vi "GUID Lookup.vi"() -> ()   [LabVIEW 2019, in "Ghost Bus Addon Shared.lvlib"]
doc: "Use this Global VI to access the GUIDs assigned to the page resources of the Custom Device."
uses:
  Ghost Bus Addon Shared.lvlib
panel:
  in  "Override Channel Page Name":string="Override"
  in  "Data Channel Page Name":string="Data"
  in  "Override Frames Page Name":string="Override Frames"
  in  "Override Frames GUID":string="6DBD21E7-9AC1-4A33-BA91-2620717C270E"
  in  "On Compile Settings":string="On Compile Settings"
  in  "Override Signal GUID":string="A0DBE684-75DE-40FF-ABFB-257FA9974665"
  in  "Data Signal GUID":string="10435930-D9E5-4765-86ED-FFE3B81430E0"
  in  "Frame.ID":string="XNET.Primary.LoopPriority"
  in  "XNET.Ghost.FDISOMode":string="XNET.Ghost.FDISOMode"
  in  "XNET.Ghost.LoopPriority":string="XNET.Ghost.LoopPriority"
  in  "XNET.Ghost.IOMode":string="XNET.Ghost.IOMode"
  in  "XNET.Ghost.FDRate":string="XNET.Ghost.FDRate"
  in  "XNET.Ghost.Termination":string="XNET.Ghost.Termination"
  in  "XNET.Ghost.Rate":string="XNET.Ghost.Rate"
  in  "XNET.Ghost.Port":string="XNET.Ghost.Port"
  in  "To Primary Bus Page Name":string="To Primary Bus"
  in  "To Ghost Bus Page Name":string="To Ghost Bus"
  in  "Settings Page Name":string="Settings"
  in  "Enable Page Name":string="Enable"
  in  "Enable Channel GUID":string="6B6F940E-5E79-447D-84E5-02DD399E6370"
  in  "Settings GUID":string="9EFE9432-3035-4F22-AD7D-DDC55D3B893F"
  in  "To Primary Bus GUID":string="F56B78C2-8EF9-4685-942E-B770392E4C5B"
  in  "To Ghost Bus GUID":string="7467F215-F187-4AC4-A182-357DF27361BD"
  in  "Override Frame GUID":string="3D195969-2661-40C8-A580-19595CD6B5C5"
  in  "Status Channel GUID":string="1C67F462-1B2F-4305-AD9C-25DD02EFA2E8"
  in  "Status GUID":string="8E6559CC-D8D1-4FEC-967E-A75255AC33F0"
  in  "Status Page Name":string="Status"
  in  "Status.Duration":string="Duration"
  in  "Status.ErrorStatus":string="Error Code"
  in  "Status.Period":string="Period"
  in  "XNET.Primary.FDISOMode":string="XNET.Primary.FDISOMode"
  in  "XNET.Primary.LoopPriority":string="XNET.Primary.LoopPriority"
  in  "XNET.Primary.IOMode":string="XNET.Primary.IOMode"
  in  "XNET.Primary.FDRate":string="XNET.Primary.FDRate"
  in  "XNET.Primary.Termination":string="XNET.Primary.Termination"
  in  "XNET.Primary.Rate":string="XNET.Primary.Rate"
  in  "XNET.Primary.Port":string="XNET.Primary.Port"
  in  "XNET.Cluster":string="XNET.Cluster"
  in  "XNET.Database":string="XNET.Database"
  in  "Help.FileName":string="Ghost Bus Addon.chm"
  out "Error Codes":cluster{"number":i32, "trimmed string":string}[](array[cluster])=[{"number"=0, "trimmed string"="<0> No Error."}, {"number"=-1074384895, "trimmed string"="<-1074384895> An internal error occurred in the NI-XNET driver."}, {"number"=-1074384894, "trimmed string"="<-1074384894> Board self test failed(code 2)."}, {"number"=-1074384893, "trimmed string"="<-1074384893> Board self test failed(code 3)."}, {"number"=-1074384892, "trimmed string"="<-1074384892> Board self test failed(code 4)."}, {"number"=-1074384891, "trimmed string"="<-1074384891> Board self test failed(code 5)."}, {"number"=-1074384890, "trimmed string"="<-1074384890> Board self test failed(code 6)."}, {"number"=-1074384889, "trimmed string"="<-1074384889> Computer went to hibernation mode and the board lost power."}, {"number"=-1074384888, "trimmed string"="<-1074384888> A write queue overflowed."}, {"number"=-1074384887, "trimmed string"="<-1074384887> The board's firmware did not answer a command."}, {"number"=-1074384886, "trimmed string"="<-1074384886> The operation timed out."}, {"number"=-1074384885, "trimmed string"="<-1074384885> A read queue overflowed."}, {"number"=-1074384884, "trimmed string"="<-1074384884> The Read buffer is too small to hold a single frame."}, {"number"=-1074384883, "trimmed string"="<-1074384883> You tried to open the same frame twice."}, {"number"=-1074384882, "trimmed string"="<-1074384882> You tried to open the same stream object twice."}, {"number"=-1074384881, "trimmed string"="<-1074384881> Self test is not possible since the board is in use by an application."}, {"number"=-1074384880, "trimmed string"="<-1074384880> Allocation of memory failed."}, {"number"=-1074384879, "trimmed string"="<-1074384879> The maximum number of sessions was exceeded."}, {"number"=-1074384878, "trimmed string"="<-1074384878> The maximum number of sessions has been exceeded."}, {"number"=-1074384877, "trimmed string"="<-1074384877> The maximum number of devices has been detected."}, {"number"=-1074384876, "trimmed string"="<-1074384876> A driver support file is missing."}, {"number"=-1074384875, "trimmed string"="<-1074384875> This indicates that a NULL pointer or an empty string was passed to a function."}, {"number"=-1074384874, "trimmed string"="<-1074384874> The maximum number of schedules has been detected."}, {"number"=-1074384873, "trimmed string"="<-1074384873> Board self test failed (code 17)."}, {"number"=-1074384872, "trimmed string"="<-1074384872> You cannot start an NI-XNET application while a self test is in progress."}, {"number"=-1074384864, "trimmed string"="<-1074384864> An invalid reference has been passed to a NI-XNET session function."}, {"number"=-1074384863, "trimmed string"="<-1074384863> An invalid reference has been passed to a NI-XNET system function."}, {"number"=-1074384862, "trimmed string"="<-1074384862> A device reference was expected for a NI-XNET session function."}, {"number"=-1074384861, "trimmed string"="<-1074384861> An interface reference was expected for a NI-XNET session function."}, {"number"=-1074384860, "trimmed string"="<-1074384860> You have configured a property that conflicts with the current mode of the session."}, {"number"=-1074384859, "trimmed string"="<-1074384859> The XNET Create Timing Source VI is supported only on LabVIEW Real-Time targets currently running the Phar Lap ETS Real-Time Operating System."}, {"number"=-1074384858, "trimmed string"="<-1074384858> You tried to create more than one LabVIEW timing source for a single interface."}, {"number"=-1074384857, "trimmed string"="<-1074384857> You invoked two or more VIs simultaneously for the same session, and those VIs do not support overlap."}, {"number"=-1074384856, "trimmed string"="<-1074384856> You are trying to start an interface that is missing bus power for the transceiver."}, {"number"=-1074384855, "trimmed string"="<-1074384855> The connection with a CompactDAQ chassis was lost, and the host software and modules are out of sync."}, {"number"=-1074384783, "trimmed string"="<-1074384783> The transceiver value set is invalid (for this port, e.g., LS on a HS port) or you are trying to perform an operation that requires a different transceiver (e.g., trying to change the state of a disconnected transceiver)."}, {"number"=-1074384782, "trimmed string"="<-1074384782> The baud rate value set is invalid."}, {"number"=-1074384781, "trimmed string"="<-1074384781> No baud rate value has been set."}, {"number"=-1074384780, "trimmed string"="<-1074384780> The bit timing values set are invalid."}, {"number"=-1074384779, "trimmed string"="<-1074384779> The baud rate set does not match the transceiver's allowed range."}, {"number"=-1074384778, "trimmed string"="<-1074384778> The configured terminal is not known for this interface."}, {"number"=-1074384777, "trimmed string"="<-1074384777> The configured terminal is inappropriate for the hardware."}, {"number"=-1074384776, "trimmed string"="<-1074384776> The source that you connected to the Master Timebase destination is missing."}, {"number"=-1074384775, "trimmed string"="<-1074384775> The source that you connected to the Master Timebase destination is not generating an appropriate signal."}, {"number"=-1074384774, "trimmed string"="<-1074384774> You are trying to disconnect a synchronization terminal that is not currently connected."}, {"number"=-1074384773, "trimmed string"="<-1074384773> You are trying to connect a synchronization terminal that is already in use."}, {"number"=-1074384772, "trimmed string"="<-1074384772> You are trying to connect an XNET terminal as a source terminal,  but the desired XNET terminal is not valid as a source terminal."}, {"number"=-1074384771, "trimmed string"="<-1074384771> You are trying to connect an XNET terminal as a destination terminal, but the desired XNET terminal is not valid as a destination terminal."}, {"number"=-1074384770, "trimmed string"="<-1074384770> You are trying to connect two XNET terminals that are incompatible."}, {"number"=-1074384769, "trimmed string"="<-1074384769> The source that you connected to the Master Timebase destination has disappeared."}, {"number"=-1074384768, "trimmed string"="<-1074384768> You called Read (State : FlexRay : Cycle Macrotick), and the FlexRay Macrotick is not connected as the master timebase of the interface."}, {"number"=-1074384767, "trimmed string"="<-1074384767> The database specified could not be opened."}, {"number"=-1074384766, "trimmed string"="<-1074384766> The cluster was not found in the database."}, {"number"=-1074384765, "trimmed string"="<-1074384765> The frame was not found in the database."}, {"number"=-1074384764, "trimmed string"="<-1074384764> The signal was not found in the database."}, {"number"=-1074384763, "trimmed string"="<-1074384763> A necessary property for a cluster was not found in the database."}, {"number"=-1074384762, "trimmed string"="<-1074384762> A necessary property for a frame was not found in the database."}, {"number"=-1074384761, "trimmed string"="<-1074384761> A necessary property for a signal was not found in the database."}, {"number"=-1074384760, "trimmed string"="<-1074384760> Multiple clusters have been specified in one session, either directly (Stream I/O), or through the signals or frames specified."}, {"number"=-1074384759, "trimmed string"="<-1074384759> You specified a database of ':subordinate:' for a session mode other than mode of Frame Input Stream."}, {"number"=-1074384758, "trimmed string"="<-1074384758> The interface name given does not specify a valid and existing interface."}, {"number"=-1074384757, "trimmed string"="<-1074384757> The operation is invalid for this interface (e.g., you tried to open a set of FlexRay frames on a CAN interface, or tried to request a CAN property from a FlexRay interface)."}, {"number"=-1074384756, "trimmed string"="<-1074384756> You tried to set the AutoStart property to FALSE for an Input session."}, {"number"=-1074384755, "trimmed string"="<-1074384755> The property ID you specified is not valid (or not valid for the current session mode or form factor)."}, {"number"=-1074384754, "trimmed string"="<-1074384754> The contents of the property is bigger than the size specified."}, {"number"=-1074384753, "trimmed string"="<-1074384753> The function you called is not defined for the session mode (e.g., you called a frame I/O function on a signal I/O session)."}, {"number"=-1074384752, "trimmed string"="<-1074384752> The data that you passed to XNET Write or XNET Read is too small to hold all the data specified for the session."}, {"number"=-1074384751, "trimmed string"="<-1074384751> For Signal Output sessions, the multiplexer signals used in the session must be specified explicitly in the signal list."}, {"number"=-1074384750, "trimmed string"="<-1074384750> You used an XNET Session IO name, and that session was not found in your LabVIEW project."}, {"number"=-1074384749, "trimmed string"="<-1074384749> You used the same XNET session name in multiple top-level VIs, which is not supported."}, {"number"=-1074384748, "trimmed string"="<-1074384748> To execute this function properly, the session's list must contain only one frame."}, {"number"=-1074384747, "trimmed string"="<-1074384747> You used the same alias for different database files which is not allowed."}, {"number"=-1074384746, "trimmed string"="<-1074384746> You try to deploy a database file while another deployment is in progress."}, {"number"=-1074384745, "trimmed string"="<-1074384745> A signal or frame session has been opened, but it does not contain signals or frames."}, {"number"=-1074384744, "trimmed string"="<-1074384744> The session mode selected is not supported by the protocol of the specified interface."}, {"number"=-1074384743, "trimmed string"="<-1074384743> A session was created by references, but no database references have been specified."}, {"number"=-1074384742, "trimmed string"="<-1074384742> The interface has already been opened with different cluster settings than the ones specified for this session."}, {"number"=-1074384741, "trimmed string"="<-1074384741> The cycle repetition of a frame in the database for the FlexRay protocol is invalid."}, {"number"=-1074384740, "trimmed string"="<-1074384740> You called XNET Clear for the session, then tried to perform another operation."}, {"number"=-1074384739, "trimmed string"="<-1074384739> You called Create Session VI with a list of items that does not match the mode."}, {"number"=-1074384738, "trimmed string"="<-1074384738> You tried to create a new session while the interface is already running."}, {"number"=-1074384737, "trimmed string"="<-1074384737> You wrote a frame whose payload length is larger than the maximum payload allowed by the database (e.g., wrote 10 bytes for CAN frame, max 8 bytes)."}, {"number"=-1074384736, "trimmed string"="<-1074384736> You called a Read function with a nonzero timeout, and you used a negative numberToRead."}, {"number"=-1074384735, "trimmed string"="<-1074384735> Timestamps are not (yet) supported for Write Signal XY."}, {"number"=-1074384734, "trimmed string"="<-1074384734> The condition parameter passed to Wait is not known."}, {"number"=-1074384733, "trimmed string"="<-1074384733> You attempted an I/O operation, but the session is not yet started (and the AutoStart property is set to FALSE)."}, {"number"=-1074384732, "trimmed string"="<-1074384732> The maximum number of Wait operations has been exceeded."}, {"number"=-1074384731, "trimmed string"="<-1074384731> You used an invalid name for an XNET Device."}, {"number"=-1074384730, "trimmed string"="<-1074384730> A terminal name passed to ConnectTerminals or DisconnectTerminals is unknown."}, {"number"=-1074384729, "trimmed string"="<-1074384729> You tried to blink the port LEDs but these are currently busy."}, {"number"=-1074384728, "trimmed string"="<-1074384728> You tried to set a FlexRay keyslot ID that is not listed as valid in the database."}, {"number"=-1074384727, "trimmed string"="<-1074384727> You tried to set a queue size that is bigger than the maximum allowed."}, {"number"=-1074384726, "trimmed string"="<-1074384726> You wrote a frame whose payload length is different than the payload length configured by the database."}, {"number"=-1074384725, "trimmed string"="<-1074384725> The index to indicate an session list element is too large."}, {"number"=-1074384724, "trimmed string"="<-1074384724> You have tried to create a session that is invalid for the mode of the driver/firmware."}, {"number"=-1074384723, "trimmed string"="<-1074384723> The trigger signal for a frame is allowed only in Single Point Signal sessions (Input or Output)."}, {"number"=-1074384722, "trimmed string"="<-1074384722> To execute this function properly, the session's list must contain only one cluster."}, {"number"=-1074384721, "trimmed string"="<-1074384721> You attempted to convert a CAN or LIN frame with a payload length greater than 8."}, {"number"=-1074384720, "trimmed string"="<-1074384720> Allocation of memory failed for the data returned from LabVIEW XNET Read."}, {"number"=-1074384719, "trimmed string"="<-1074384719> Allocation of memory failed in the firmware."}, {"number"=-1074384718, "trimmed string"="<-1074384718> The NI-XNET driver no longer can communicate with the device."}, {"number"=-1074384717, "trimmed string"="<-1074384717> A LIN schedule has an invalid priority."}, {"number"=-1074384716, "trimmed string"="<-1074384716> (Dis)ConnectTerminals is not allowed for XNET C Series modules."}, {"number"=-1074384715, "trimmed string"="<-1074384715> You requested a time (like Start or Communication Time) before the event has happened."}, {"number"=-1074384714, "trimmed string"="<-1074384714> An internal input queue overflowed."}, {"number"=-1074384713, "trimmed string"="<-1074384713> A bad firmware image file can not be loaded to the hardware."}, {"number"=-1074384712, "trimmed string"="<-1074384712> The encoding of embedded network data (CAN, FlexRay, LIN, etc.) within the TDMS file is invalid."}, {"number"=-1074384711, "trimmed string"="<-1074384711> The NI-XNET hardware no longer can communicate with the transceiver cable."}, {"number"=-1074384710, "trimmed string"="<-1074384710> The NI-XNET driver timed out when performing low-level communication with the device."}, {"number"=-1074384709, "trimmed string"="<-1074384709> A transfer to the C Series module was aborted."}, {"number"=-1074384708, "trimmed string"="<-1074384708> An invalid value has been specified for the CAN FD ISO Mode."}, {"number"=-1074384704, "trimmed string"="<-1074384704> A property value was out of range or incorrect."}, {"number"=-1074384703, "trimmed string"="<-1074384703> Integration of the interface into the FlexRay cluster failed, so communication did not start for the interface."}, {"number"=-1074384688, "trimmed string"="<-1074384688> The PDU was not found in the database."}, {"number"=-1074384687, "trimmed string"="<-1074384687> A necessary property for a PDU was not found in the database."}, {"number"=-1074384686, "trimmed string"="<-1074384686> You tried to open the same PDU twice."}, {"number"=-1074384685, "trimmed string"="<-1074384685> You can access this database object only by PDU, not by frame."}, {"number"=-1074384640, "trimmed string"="<-1074384640> Remote communication with the LabVIEW RT target failed."}, {"number"=-1074384639, "trimmed string"="<-1074384639> File transfer communication with the LabVIEW Real-Time (RT) target failed."}, {"number"=-1074384638, "trimmed string"="<-1074384638> File transfer to the LabVIEW Real-Time (RT) target failed, because the required files could not be accessed."}, {"number"=-1074384637, "trimmed string"="<-1074384637> The database file you want to use is already assigned to another alias."}, {"number"=-1074384636, "trimmed string"="<-1074384636> An internal file used by NI-XNET could not be accessed."}, {"number"=-1074384635, "trimmed string"="<-1074384635> The file cannot be deployed because another file deployment is already active."}, {"number"=-1074384617, "trimmed string"="<-1074384617> The nixnet.dll or one of its components could not be loaded."}, {"number"=-1074384610, "trimmed string"="<-1074384610> You attempted to perform an action on a session or interface that is started, and the action that requires the session/interface to be stopped."}, {"number"=-1074384609, "trimmed string"="<-1074384609> You have passed a default payload to the firmware where the number of bytes in the payload is larger than the number of bytes that this frame can transmit."}, {"number"=-1074384605, "trimmed string"="<-1074384605> You attempted to set a CAN arbitration ID with an invalid value."}, {"number"=-1074384604, "trimmed string"="<-1074384604> You attempted to set a LIN ID with an invalid value."}, {"number"=-1074384592, "trimmed string"="<-1074384592> Too many open files."}, {"number"=-1074384591, "trimmed string"="<-1074384591> Bad reference has been passed to a database function, e.g., a session reference, or frame reference to retrieve properties from a signal."}, {"number"=-1074384590, "trimmed string"="<-1074384590> Creating a database file failed."}, {"number"=-1074384589, "trimmed string"="<-1074384589> A cluster with the same name already exists in the database."}, {"number"=-1074384588, "trimmed string"="<-1074384588> A frame with the same name already exists in the cluster."}, {"number"=-1074384587, "trimmed string"="<-1074384587> A signal with the same name already exists in the frame."}, {"number"=-1074384586, "trimmed string"="<-1074384586> An ECU with the same name already exists in the cluster."}, {"number"=-1074384585, "trimmed string"="<-1074384585> A subframe with the same name already exists in the frame."}, {"number"=-1074384584, "trimmed string"="<-1074384584> The operation is improper for the protocol in use, e.g., you cannot assign FlexRay channels to a CAN frame."}, {"number"=-1074384583, "trimmed string"="<-1074384583> Wrong parent relationship for a child that you are creating with XNET Database Create."}, {"number"=-1074384581, "trimmed string"="<-1074384581> The retrieved required property is not defined on the specified object."}, {"number"=-1074384580, "trimmed string"="<-1074384580> The feature is not supported under LabVIEW RT, e.g.Save Database"}, {"number"=-1074384579, "trimmed string"="<-1074384579> The object name contains unsupported characters."}, {"number"=-1074384578, "trimmed string"="<-1074384578> Unsupported database format."}, {"number"=-1074384577, "trimmed string"="<-1074384577> Database object not found (e.g., an object with given name does not exist)."}, {"number"=-1074384576, "trimmed string"="<-1074384576> Database cache file cannot be removed or replaced on the disc (e.g., file is write-protected)."}, {"number"=-1074384575, "trimmed string"="<-1074384575> You are trying to write a read-only property, e.g., the mux value on a signal is a read only property (can be changed on the subframe)."}, {"number"=-1074384574, "trimmed string"="<-1074384574> You are trying to change a signal to be a mux signal, but a mux is already defined in this frame"}, {"number"=-1074384572, "trimmed string"="<-1074384572> You are trying to define FlexRay in-cycle-repetition slots before defining the first slot."}, {"number"=-1074384571, "trimmed string"="<-1074384571> You are trying to define FlexRay in-cycle-repetition channels before defining the first channels."}, {"number"=-1074384570, "trimmed string"="<-1074384570> You must define the protocol before setting this property (e.g., the frame ID has a different meaning in a CAN or FlexRay cluster)."}, {"number"=-1074384569, "trimmed string"="<-1074384569> The database information on the real-time system has been created with an older NI-XNET version."}, {"number"=-1074384568, "trimmed string"="<-1074384568> Frame ConfigStatus: A signal within the frame exceeds the frame boundaries (Payload Length)."}, {"number"=-1074384567, "trimmed string"="<-1074384567> Frame ConfigStatus: A signal within the frame overlaps another signal."}, {"number"=-1074384566, "trimmed string"="<-1074384566> Frame ConfigStatus: A integer signal within the frame is defined with more than 52 bits."}, {"number"=-1074384565, "trimmed string"="<-1074384565> Frame ConfigStatus: Frame is defined with an invalid payload size."}, {"number"=-1074384564, "trimmed string"="<-1074384564> You are trying to add transmitted FlexRay frames to an ECU, with at least two of them having Startup or Sync property on."}, {"number"=-1074384563, "trimmed string"="<-1074384563> You are trying to add TX/RX frames to an ECU which are defined in a different cluster than the ECU."}, {"number"=-1074384562, "trimmed string"="<-1074384562> Database name parameter is incorrect."}, {"number"=-1074384561, "trimmed string"="<-1074384561> Database object is locked because it is used in a session."}, {"number"=-1074384560, "trimmed string"="<-1074384560> Alias name passed to a function is not defined."}, {"number"=-1074384559, "trimmed string"="<-1074384559> Database file cannot be saved because frames are assigned to FlexRay channels not defined in the cluster."}, {"number"=-1074384558, "trimmed string"="<-1074384558> Frame ConfigStatus: This FlexRay frame transmitted in a dynamic segment uses both channels A and B."}, {"number"=-1074384557, "trimmed string"="<-1074384557> Database is locked because it is being modified by an another instance of the same application."}, {"number"=-1074384556, "trimmed string"="<-1074384556> A frame name is ambiguous (e.g., a frame with the same name exists in another cluster)."}, {"number"=-1074384555, "trimmed string"="<-1074384555> A signal name is ambiguous (e.g., a signal with the same name exists in another frame)."}, {"number"=-1074384554, "trimmed string"="<-1074384554> An ECU name is ambiguous (e.g., an ECU with the same name exists in another cluster)."}, {"number"=-1074384553, "trimmed string"="<-1074384553> A subframe name is ambiguous (e.g., a subframe with the same name exists in another cluster)."}, {"number"=-1074384552, "trimmed string"="<-1074384552> A LIN schedule name is ambiguous (e.g., a schedule with the same name exists in another cluster)."}, {"number"=-1074384551, "trimmed string"="<-1074384551> A LIN schedule with the same name already exists in the database."}, {"number"=-1074384550, "trimmed string"="<-1074384550> Multiplexers (mode-dependent signals) are not supported when the given protocol is used."}, {"number"=-1074384549, "trimmed string"="<-1074384549> Saving a FIBEX file containing a LIN cluster is not supported in this NI-XNET version."}, {"number"=-1074384548, "trimmed string"="<-1074384548> This property requires an ECU configured as LIN master to be present in this cluster."}, {"number"=-1074384547, "trimmed string"="<-1074384547> You have tried to create a session using a frame that is incompatible with the selected session type."}, {"number"=-1074384546, "trimmed string"="<-1074384546> You cannot mix open of NI-XNET database objects as both manual and automatic."}, {"number"=-1074384545, "trimmed string"="<-1074384545> Due to problems in LabVIEW versions 8.5 through 8.6.1, automatic open of NI-XNET database objects is not supported."}, {"number"=-1074384544, "trimmed string"="<-1074384544> You called a Write function with the number of array elements (frames or signals) different than the number of elements configured in the session (such as the \"list\" parameter of the Create Session function)."}, {"number"=-1074384543, "trimmed string"="<-1074384543> You used XNET session from multiple LabVIEW projects (or multiple executables), which NI-XNET does not support."}, {"number"=-1074384542, "trimmed string"="<-1074384542> When an XNET session is used at runtime, all sessions in the same scope are created on the interface."}, {"number"=-1074384541, "trimmed string"="<-1074384541> You used an empty name for an XNET database object (database, cluster, ECU, frame, or signal)."}, {"number"=-1074384540, "trimmed string"="<-1074384540> You used a name for an XNET database object (such as frame or signal) that did not include a valid cluster selection."}, {"number"=-1074384539, "trimmed string"="<-1074384539> Unsupported database file version."}, {"number"=-1074384538, "trimmed string"="<-1074384538> You used an empty name for the XNET Session."}, {"number"=-1074384537, "trimmed string"="<-1074384537> There is not enough message RAM on the FlexRay hardware to configure the data partition for the object(s)."}, {"number"=-1074384536, "trimmed string"="<-1074384536> The FlexRay keyslot ID has been configured and a startup session has been created."}, {"number"=-1074384535, "trimmed string"="<-1074384535> An unsupported session was created."}, {"number"=-1074384528, "trimmed string"="<-1074384528> An XNET session was created after starting the Interface."}, {"number"=-1074384527, "trimmed string"="<-1074384527> The Single Slot property was enabled on the XNET FlexRay Interface after the interface had started."}, {"number"=-1074384526, "trimmed string"="<-1074384526> The FlexRay macrotick offset specified for XNET Create Timing Source is unsupported."}, {"number"=-1074384525, "trimmed string"="<-1074384525> You used invalid syntax in the name of a database object (signal, frame, or ECU)."}, {"number"=-1074384524, "trimmed string"="<-1074384524> A LIN schedule entry name is ambiguous, e.g., a schedule entry with the same name exists in another schedule."}, {"number"=-1074384523, "trimmed string"="<-1074384523> A LIN schedule entry with the same name already exists in the schedule."}, {"number"=-1074384522, "trimmed string"="<-1074384522> At least one of the frames in the session has an undefined identifier."}, {"number"=-1074384521, "trimmed string"="<-1074384521> At least one of the frames in the session has an undefined payload length."}, {"number"=-1074384520, "trimmed string"="<-1074384520> At least one of the signals in the session has an undefined start bit."}, {"number"=-1074384519, "trimmed string"="<-1074384519> At least one of the signals in the session has an undefined number of bits."}, {"number"=-1074384518, "trimmed string"="<-1074384518> At least one of the signals in the session has an undefined byte order."}, {"number"=-1074384517, "trimmed string"="<-1074384517> At least one of the signals in the session has an undefined data type."}, {"number"=-1074384516, "trimmed string"="<-1074384516> At least one of the subframes in the session has an undefined multiplexer value."}, {"number"=-1074384515, "trimmed string"="<-1074384515> You provided an invalid index to Write (State LIN Schedule Change)."}, {"number"=-1074384514, "trimmed string"="<-1074384514> You provided an invalid name to Write (State LIN Schedule Change)."}, {"number"=-1074384513, "trimmed string"="<-1074384513> You provided an invalid active index for the session property.\nFor LabVIEW, this is the Frame:Active in the session property node.\nFor C/C++, this is the ActiveIndex parameter of nxGetSubProperty/nxSetSubProperty."}, {"number"=-1074384512, "trimmed string"="<-1074384512> You provided an invalid name for Frame:Active of the session property node."}, {"number"=-1074384511, "trimmed string"="<-1074384511> The database you are using requires using PDUs, and the operation is ambiguous with respect to PDUs."}, {"number"=-1074384510, "trimmed string"="<-1074384510> A PDU with the same name already exists in the cluster."}, {"number"=-1074384509, "trimmed string"="<-1074384509> You are trying to assign start bits or update bits to PDUs referenced in a frame, but the number of elements in this array is different than the number of referenced PDUs."}, {"number"=-1074384508, "trimmed string"="<-1074384508> The configuration of this object requires using advanced PDUs, which the given protocol does not support."}, {"number"=-1074384507, "trimmed string"="<-1074384507> The maximum number of PDUs has been exceeded."}, {"number"=-1074384506, "trimmed string"="<-1074384506> This mode value is not currently supported."}, {"number"=-1074384505, "trimmed string"="<-1074384505> The firmware image on your XNET hardware is corrupted."}, {"number"=-1074384504, "trimmed string"="<-1074384504> The firmware version of your XNET hardware is not in sync with your host computer."}, {"number"=-1074384503, "trimmed string"="<-1074384503> The firmware version of your XNET C Series module is not in sync with the NI-XNET software on your remote target."}, {"number"=-1074384502, "trimmed string"="<-1074384502> The terminal you are trying to use is already in use."}, {"number"=-1074384501, "trimmed string"="<-1074384501> You need to install a supported version of NI-DAQmx for your XNET C Series module to work correctly with your Compact DAQ system."}, {"number"=-1074384500, "trimmed string"="<-1074384500> Unable to create the requested route."}, {"number"=-1074384499, "trimmed string"="<-1074384499> You attempted to transmit a go to sleep frame (by setting the LIN Sleep mode to Remote Sleep) on a LIN interface configured as slave."}, {"number"=-1074384498, "trimmed string"="<-1074384498> You attempted to set properties related to Sleep and Wakeup when the FlexRay cluster defined in the Fibex file does not support it."}, {"number"=-1074384497, "trimmed string"="<-1074384497> A LIN diagnostic schedule change requires the diagnostic schedule to be defined in the database."}, {"number"=-1074384494, "trimmed string"="<-1074384494> The data payload written for a diagnostic frame for transmit does not conform to the LIN transport layer specification."}, {"number"=-1074384493, "trimmed string"="<-1074384493> An error occurred within the NI-XNET example code for logfile access (TDMS)."}, {"number"=-1074384384, "trimmed string"="<-1074384384> You attempted to write a LIN schedule and use a stream output replay timing mode concurrently."}, {"number"=-1074384383, "trimmed string"="<-1074384383> You attempted to create a session that is incompatible with the LIN interface personality (master or slave), or set the LIN interface personality to one that is incompatible with a session already created for it."}, {"number"=-1074384382, "trimmed string"="<-1074384382> You attempted to save an LDF or DBC database, but the passed reference is not a database cluster."}, {"number"=-1074384381, "trimmed string"="<-1074384381> You tried to assign the same interface name twice."}, {"number"=-1074384380, "trimmed string"="<-1074384380> Transceiver cable hardware revision is too new."}, {"number"=-1074384379, "trimmed string"="<-1074384379> Transceiver cable image revision is too new."}, {"number"=-1074384378, "trimmed string"="<-1074384378> The property does not apply to this type of hardware."}, {"number"=-1074384377, "trimmed string"="<-1074384377> Exporting cluster into the specified database type failed."}, {"number"=-1074384376, "trimmed string"="<-1074384376> A J1939 input queue overflowed."}, {"number"=-1074384375, "trimmed string"="<-1074384375> You are trying to transmit a non-J1939 frame with more than 8 bytes."}, {"number"=-1074384374, "trimmed string"="<-1074384374> You are trying to transmit a J1939 frame, but no J1939 address is assigned to the session."}, {"number"=-1074384373, "trimmed string"="<-1074384373> The received J1939 TP.CM_CTS message has the wrong total size."}, {"number"=-1074384372, "trimmed string"="<-1074384372> The next packet value of the received J1939 TP.CM_CTS message is larger than the total number of packets."}, {"number"=-1074384371, "trimmed string"="<-1074384371> The received J1939 TP.CM_CTS message has a number of packets of 0, but the next packet number is not 255."}, {"number"=-1074384370, "trimmed string"="<-1074384370> The received J1939 TP.CM_CTS message has a next packet value of 0."}, {"number"=-1074384369, "trimmed string"="<-1074384369> The received J1939 TP.CM_CTS message does not have the same PGN as in the TP.CM_RTS message."}, {"number"=-1074384368, "trimmed string"="<-1074384368> Received unexpected sequence number in the J1939 TP.DT message."}, {"number"=-1074384367, "trimmed string"="<-1074384367> More Packets are requested than allowed in the J1939 TP.CM_CTS message."}, {"number"=-1074384366, "trimmed string"="<-1074384366> J1939 Timeout T1 while waiting for data."}, {"number"=-1074384365, "trimmed string"="<-1074384365> J1939 Timeout T2 while waiting for data."}, {"number"=-1074384364, "trimmed string"="<-1074384364> J1939 Timeout T3 while waiting for TP.CM_CTS or TP.CM_EndOfMsgAck."}, {"number"=-1074384363, "trimmed string"="<-1074384363> J1939 Timeout T4 while waiting for next CTS MSG."}, {"number"=-1074384362, "trimmed string"="<-1074384362> Received wrong DLC in the J1939 TP.CM_RTS message."}, {"number"=-1074384361, "trimmed string"="<-1074384361> Received wrong DLC in the J1939 TP.CM_CTS message."}, {"number"=-1074384360, "trimmed string"="<-1074384360> Received wrong DLC in the J1939 TP.CM_BAM message."}, {"number"=-1074384359, "trimmed string"="<-1074384359> Received wrong DLC in the J1939 TP.DT message."}, {"number"=-1074384358, "trimmed string"="<-1074384358> Received wrong DLC in the J1939 TP.CM_Abort message."}, {"number"=-1074384357, "trimmed string"="<-1074384357> Received wrong DLC in the J1939 TP.CM_EndOfMsgAck message."}, {"number"=-1074384356, "trimmed string"="<-1074384356> Received wrong PGN in the J1939 TP.CM_Abort message."}, {"number"=-1074384355, "trimmed string"="<-1074384355> Internal error occurred for send TP.CM_CTS Hold Message."}, {"number"=-1074384354, "trimmed string"="<-1074384354> Invalid total message size in J1939 TP.CM_RTS message."}, {"number"=-1074384353, "trimmed string"="<-1074384353> Total number of packets in received J1939 TP.CM_RTS message must be greater than 1."}, {"number"=-1074384352, "trimmed string"="<-1074384352> Reserved data bytes in J1939 received message are not BFF63FF."}, {"number"=-1074384351, "trimmed string"="<-1074384351> Not enough system resources for the J1939 Transport Protocol."}, {"number"=-1074384350, "trimmed string"="<-1074384350> Received J1939 TP.CM_Abort message with reason ActiveConnection: Already in one or more connection managed sessions and cannot support another."}, {"number"=-1074384349, "trimmed string"="<-1074384349> Received J1939 TP.CM_Abort message with reason NotEnoughSystemResources: System resources were needed for another task, so this connection managed session was terminated."}, {"number"=-1074384348, "trimmed string"="<-1074384348> Received J1939 TP.CM_Abort message with reason Timeout: A timeout occurred, and this is the connection abort to close the session."}, {"number"=-1074384347, "trimmed string"="<-1074384347> Received J1939 TP.CM_Abort message with reason CtsReceived: CTS messages received when data transfer is in progress."}, {"number"=-1074384346, "trimmed string"="<-1074384346> Received J1939 TP.CM_Abort message with reason MaxRetransmit: Maximum retransmit request limit reached."}, {"number"=-1074384345, "trimmed string"="<-1074384345> Remote communication with the LabVIEW RT target failed because the host and target versions of NI-XNET are different."}, {"number"=-1074384344, "trimmed string"="<-1074384344> The CAN frame I/O mode is higher than the CAN cluster  I/O mode."}, {"number"=-1074384343, "trimmed string"="<-1074384343> The current driver cannot update the firmware on your hardware."}, {"number"=-1074384342, "trimmed string"="<-1074384342> You are trying to use the CAN Transmit I/O Mode (TxIoMode) property in an unsupported interface mode."}, {"number"=-1074384341, "trimmed string"="<-1074384341> You are trying to use the XS Transceiver Cable on unsupported hardware."}, {"number"=-1074384340, "trimmed string"="<-1074384340> You are trying to use a database alias name that contains an invalid character (for example, a comma)."}, {"number"=-1074384339, "trimmed string"="<-1074384339> You are trying to use a database filepath that contains an invalid character (for example, a comma)."}, {"number"=-1074384338, "trimmed string"="<-1074384338> You are trying to use CAN FD with a non-HS/FD port."}, {"number"=-1074384337, "trimmed string"="<-1074384337> An unconditional LIN schedule entry is incorrectly configured."}, {"number"=-1074384336, "trimmed string"="<-1074384336> An event LIN schedule entry has no collision resolving schedule assigned."}, {"number"=-1074384335, "trimmed string"="<-1074384335> You have connected your USB device to a port that supports only Full Speed (USB 1.1)."}, {"number"=-1074384334, "trimmed string"="<-1074384334> You added two or more frames with different payload sizes to the same LIN event-triggered schedule entry."}, {"number"=-1074384333, "trimmed string"="<-1074384333> You added two or more frames with different checksum types to the same event-triggered schedule entry."}, {"number"=-1074384332, "trimmed string"="<-1074384332> The versions of the NI-XNET device driver and Compact RIO driver are incompatible."}, {"number"=-1074384331, "trimmed string"="<-1074384331> The module support for this slot is missing features required for the NI-XNET driver to be able to communicate with the module."}, {"number"=-1074384330, "trimmed string"="<-1074384330> The interface you have attempted to use with NI-XNET Compatibility Library is already in use by NI-XNET."}, {"number"=-1074384329, "trimmed string"="<-1074384329> The interface you have attempted to use with NI-XNET is already in use by NI-XNET Compatibility Library."}, {"number"=-1074384328, "trimmed string"="<-1074384328> Byte array signals are not allowed for this session type or function."}, {"number"=-1074384327, "trimmed string"="<-1074384327> Mixing of byte array signals and numeric signals is not allowed for this session type."}, {"number"=-1074384326, "trimmed string"="<-1074384326> Only one byte array signal is allowed for this session type or function."}, {"number"=-1074384325, "trimmed string"="<-1074384325> The feature you have attempted to use is not supported."}, {"number"=-1074384324, "trimmed string"="<-1074384324> The specified property is write-only and is therefore not readable."}, {"number"=-1074384323, "trimmed string"="<-1074384323> FPGA download is not possible because the board is in use by an application."}, {"number"=-1074384322, "trimmed string"="<-1074384322> The trigger timestamp cannot be read, because the trigger source is not connected."}, {"number"=-1074384321, "trimmed string"="<-1074384321> The trigger timestamp cannot be read, because another operation is reading the timestamp."}, {"number"=-1074384320, "trimmed string"="<-1074384320> The wait did not complete, because it was aborted."}, {"number"=-1074384319, "trimmed string"="<-1074384319> The future time trigger cannot be generated, because the trigger destination is not connected."}, {"number"=-1074384318, "trimmed string"="<-1074384318> The log file could not be created because it already exists."}, {"number"=-1074384317, "trimmed string"="<-1074384317> Could not create or replace the log file."}, {"number"=-1074384316, "trimmed string"="<-1074384316> You cannot read data using XNET Read after a session has been started with logging enabled."}, {"number"=-1074384315, "trimmed string"="<-1074384315> A problem has been detected with the firmware on the device."}, {"number"=-1074384314, "trimmed string"="<-1074384314> A write queue overflowed for a session that has not been started."}, {"number"=-1074384313, "trimmed string"="<-1074384313> The total size of the data to be transmitted is larger than the internal write queue."}, {"number"=-1074384312, "trimmed string"="<-1074384312> The requested number of packets do not fit in the current queue."}, {"number"=-1074384311, "trimmed string"="<-1074384311> You wrote a frame whose payload length is smaller than the minimum payload size allowed."}, {"number"=-1074384310, "trimmed string"="<-1074384310> The XNET endpoint on this port cannot start while the Port Mode is set to Tap."}, {"number"=-1074384309, "trimmed string"="<-1074384309> The future time trigger cannot be generated because a previously scheduled future time trigger is still pending."}, {"number"=-1074384308, "trimmed string"="<-1074384308> The desired time to generate the future time trigger has already elapsed."}, {"number"=-1074384307, "trimmed string"="<-1074384307> The network time cannot be adjusted while this clock is a slave (i.e., not grandmaster)."}, {"number"=-1074384306, "trimmed string"="<-1074384306> Output sessions must be created using an interface's endpoint path."}, {"number"=-1074384305, "trimmed string"="<-1074384305> The time protocol cannot be used while the Port Mode is set to Tap."}, {"number"=-1074384304, "trimmed string"="<-1074384304> You cannot write data while the XNET session is started and the link is down."}, {"number"=-1074384303, "trimmed string"="<-1074384303> Device reset is not possible since the board is in use by an application."}, {"number"=-1074384302, "trimmed string"="<-1074384302> You cannot start an NI-XNET application while a device reset is in progress."}, {"number"=-1074384301, "trimmed string"="<-1074384301> You wrote a frame whose frame type value is not valid."}, {"number"=-1074384300, "trimmed string"="<-1074384300> The data path you have attempted to use is already in use by another session."}, {"number"=-1074384299, "trimmed string"="<-1074384299> The timescale value is invalid."}, {"number"=-1074384298, "trimmed string"="<-1074384298> A hardware error has occurred while reading the Port MAC address."}, {"number"=-1074384297, "trimmed string"="<-1074384297> You cannot write to the Time Sync Protocol property while the Port Mode is set to Tap."}, {"number"=-1074384296, "trimmed string"="<-1074384296> The buffer is not large enough to contain the requested path."}, {"number"=-1074384295, "trimmed string"="<-1074384295> A NULL pointer or an empty string was passed when requesting a path."}, {"number"=1073098816, "trimmed string"="<1073098816> The CAN FD baud rate you supplied exceeds the capabilities the transceiver manufacturer specified."}, {"number"=1073098885, "trimmed string"="<1073098885> There is a warning from importing the database file."}, {"number"=1073098886, "trimmed string"="<1073098886> The database file has been imported, but it was not created by the XNET Editor or using the XNET API."}, {"number"=1073098887, "trimmed string"="<1073098887> The database file was not created by the XNET Editor or using the XNET API."}, {"number"=1073099057, "trimmed string"="<1073099057> Close Database returns a warning instead of an error when an invalid reference is passed to the function."}, {"number"=1073099058, "trimmed string"="<1073099058> You are retrieving signals from a frame that uses advanced PDU configuration."}]
  in  "Custom Device GUID_Disabled":string="FAA7F77A-E3DD-4739-BD52-E4C14A9D9572"
  in  "Custom Device GUID":string="F665F79A-31C5-4337-8154-8A722BDBE03B"
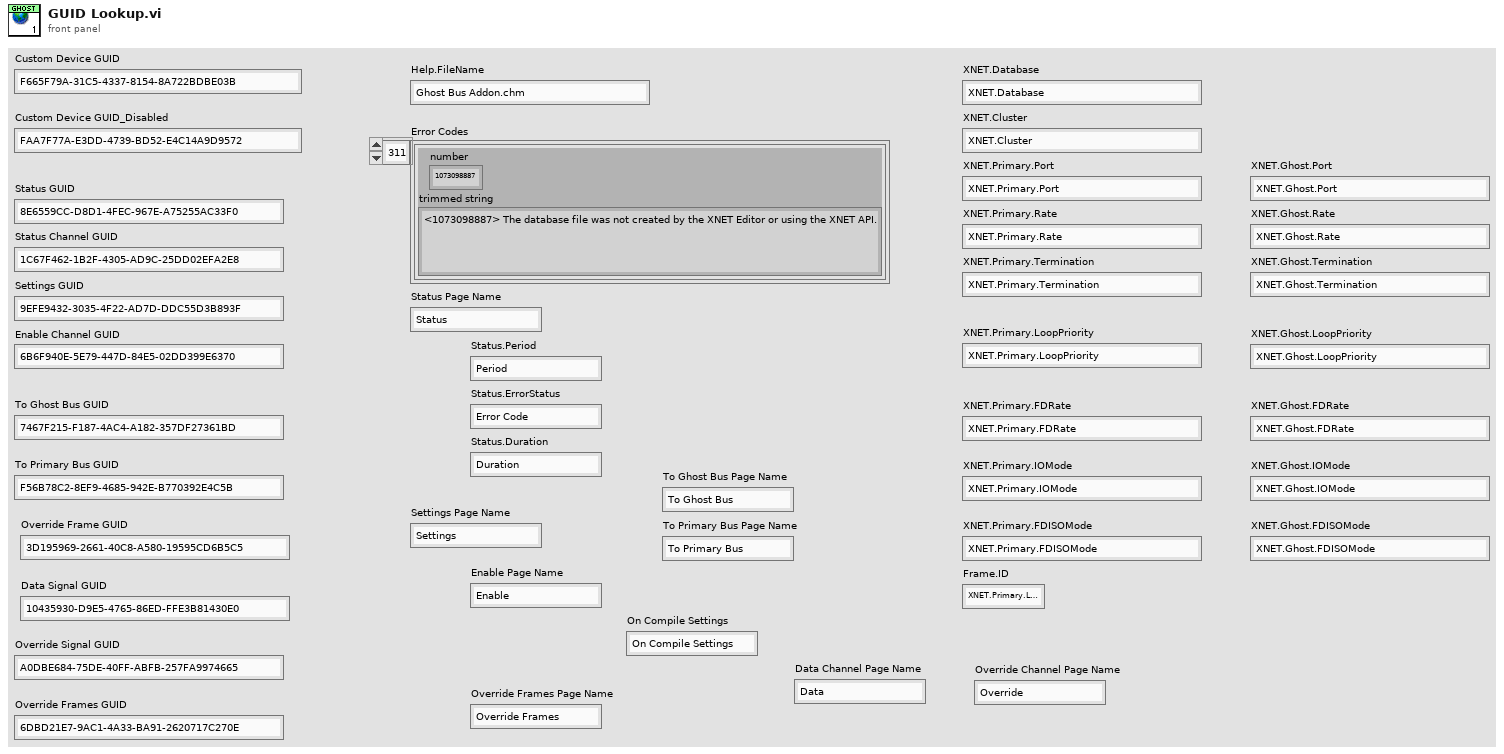
[diagram p1: front panel]
diagram:
